vi "Pracownia_6_global.vi"() -> ()   [LabVIEW 2023]
panel:
  in  "stop":bool
  out "Tablica Bitów":bool[](array[boolean])
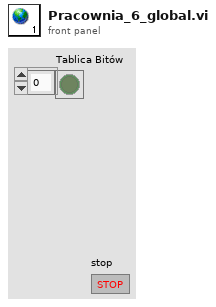
[diagram p1: front panel]
diagram:
